vi "Convert_pre_ramp_sequence.vi"(2 "Fast-seq-divider":u64, 3 "fastseq":T7(array[cluster]) {"DAC"."DAC offset" min=-1 max=0.5; "DAC"."FastChanNum" max=15 step=1; "slot#" max=4095}, 4 "Start ramp at":u64, 5 "Sequence size":u64) -> (0 "Pts to acquire":u64, 1 "Pts to keep":u64)   [LabVIEW 2013]
uses:
  Fast_sequence/sequence slot/slot-use.ctl
  Fast_sequence/sequence slot/triggers.ctl
  Fast_sequence/sequence slot/DAC.ctl
  Fast_sequence/sequence slot/DAC_fastseq-offset.ctl
  Fast_sequence/sequence slot/timing.ctl
  Fast_sequence/sequence slot/jump.ctl
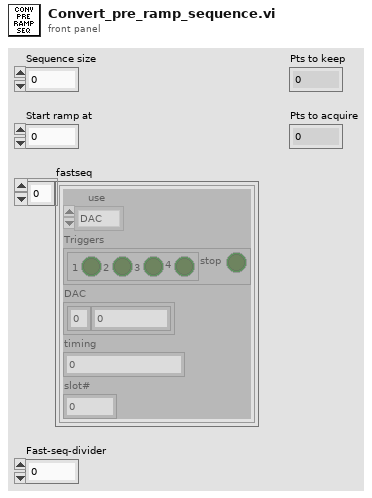
[diagram p1: front panel]
types:
  T1 = typedef "slot-use.ctl" = enum8{"DAC", "timing", "triggers", "jump"}
  T2 = typedef "triggers.ctl" = cluster{"triggers":cluster{"1":bool, "2":bool, "3":bool, "4":bool}, "stop":bool}
  T3 = typedef "DAC.ctl" = cluster{"FastChanNum":u8, "DAC offset":T4}
  T4 = typedef "DAC_fastseq-offset.ctl" = sgl
  T5 = typedef "timing.ctl" = sgl
  T6 = typedef "jump.ctl" = u16
  T7 = cluster{"use":T1, "Triggers":T2, "DAC":T3, "timing":T5, "slot#":T6}[]
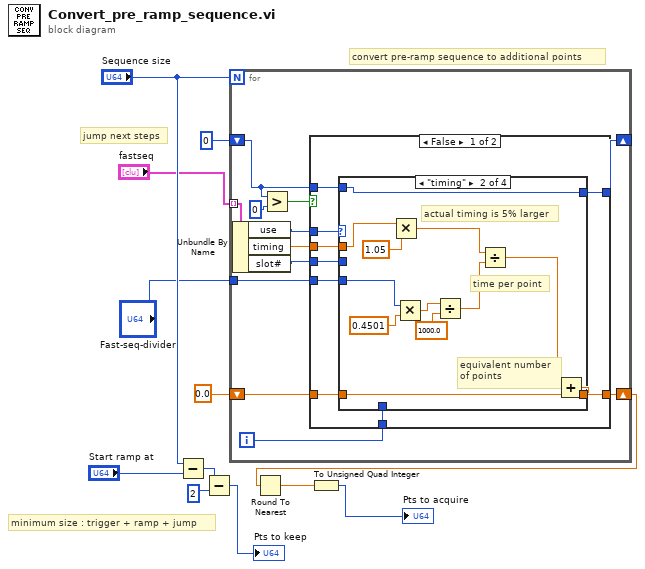
[diagram p0: block diagram]
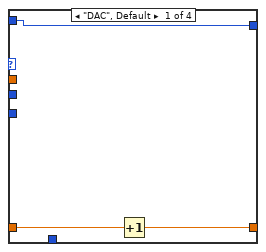
[diagram p2: hidden frame]
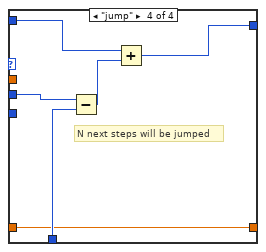
[diagram p4: hidden frame]
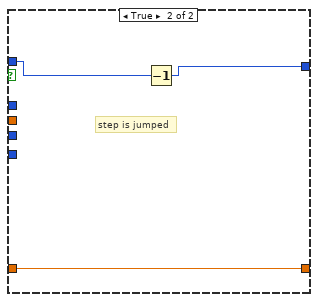
[diagram p5: hidden frame]
diagram:
  # "minimum size : trigger + ramp + jump"
  # "convert pre-ramp sequence to additional points"
  # "jump next steps"
  n1 = Subtract(x="Sequence size", y="Start ramp at") -> (x-y=w9:u64)
  n2 = Subtract(x=w9, y=2) -> (x-y=→"Pts to keep":u64)
  n3 = for {
    N: "Sequence size" -> [_]
    tunnel: "fastseq" -> [w21] mode=indexing
    shift-right: [w13] -> w5
    shift-left: 0.0 -> [w24]
    tunnel: "Fast-seq-divider" -> [w22]
    shift-right: [w18] -> _
    shift-left: 0 -> [w15]
    i -> [w17]
    n4 = Unbundle By Name(w21) -> ("use"=w23:T1, "timing"=w20:T5, "slot#"=w19:T6)
    n5 = Greater?(x=w15, y=0) -> (0:w14:bool)
    n6 = case shown="False" w14 {
      tunnel: w24 -> [w33 w57]
      tunnel: [w32 w57] -> w13
      tunnel: w23 -> [w31 _]
      tunnel: w22 -> [w30 _]
      tunnel: w20 -> [w29 _]
      tunnel: w19 -> [w28 _]
      tunnel: w15 -> [w27 w59]
      tunnel: [w26 w58] -> w18
      tunnel: w17 -> [w25 _]
      frame False {
        n7 = case shown="\"timing\"" w31 {
          tunnel: w33 -> [w36 w44 w50 w51]
          tunnel: [w35 w41 w50 w51] -> w32
          tunnel: w30 -> [_ w45 _ _]
          tunnel: w29 -> [_ w39 _ _]
          tunnel: w28 -> [_ _ _ w54]
          tunnel: w27 -> [w34 w40 w49 w56]
          tunnel: [w34 w40 w49 w55] -> w26
          tunnel: w25 -> [_ _ _ w53]
          frame "DAC", Default {
            n8 = Increment(x=w36) -> (x+1=w35:dbl)
          }
          frame "timing" {
            # "actual timing is 5% larger"
            # "equivalent number\nof points"
            # "time per point"
            n9 = Multiply(x=w39, y=1.05) -> (x*y=w38:dbl)
            n10 = Multiply(x=w45, y=0.4501) -> (x*y=w47:dbl)
            n11 = Divide(x=w47, y=1000.0) -> (x/y=w43:dbl)
            n12 = Divide(x=w38, y=w43) -> (x/y=w42:dbl)
            n13 = Add(x=w42, y=w44) -> (x+y=w41:dbl)
          }
          frame "triggers" {
            # "triggers are not\ntaken into account"
          }
          frame "jump" {
            # "N next steps will be jumped"
            n14 = Subtract(x=w54, y=w53) -> (x-y=w52:i32)
            n15 = Add(x=w56, y=w52) -> (x+y=w55:i32)
          }
        }
      }
      frame True {
        # "step is jumped"
        n16 = Decrement(x=w59) -> (x-1=w58:i32)
      }
    }
  }
  n17 = Round To Nearest(number=w5) -> (nearest integer value=w6:dbl)
  n18 = To Unsigned Quad Integer(1:w6) -> (0:→"Pts to acquire":u64)
